vi "Before Run TS.vi"(8 "error in":errorcluster, 11 "Heat Flow Test Stand in":refnum<class "Heat Flow Test Stand.lvclass">) -> (0 "error out":errorcluster, 3 "Heat Flow Test Stand out":refnum<class "Heat Flow Test Stand.lvclass">)   [LabVIEW 2019, in "Test Stands.lvlib" / "Heat Flow Test Stand.lvclass"]
uses:
  Heat Flow Test Stand.lvclass
  C:/Users/wg/Documents/LV_Projects/test-stand/App/Generic Test Stand/Generic Test Stand.lvclass
  DAC/Heat Flow/HeatFlow AIV/DAC HeatFlow AIV.lvclass
  C:/Users/wg/Documents/LV_Projects/test-stand/App/DAC/DAC.lvclass
  Results/Heat Flow Results/Heat Flow Results.lvclass
  Results/Results Method.ctl
  Generic Test Stand/Generic Test Stand.lvclass/Generic Test Stand.ctl
  Heat Flow Test Stand.lvclass/Heat Flow Test Stand.ctl
  DAC/DAC.lvclass/DAC.ctl
  Results/Heat Flow Results/Heat Flow Results.lvclass/Heat Flow Results.ctl
  DAC/DAC.lvclass
  Generic Test Stand/Generic Test Stand.lvclass
  Results/Results.lvlib
  DAC/Heat Flow/RTD Temp/DAC RTD Temp.lvclass
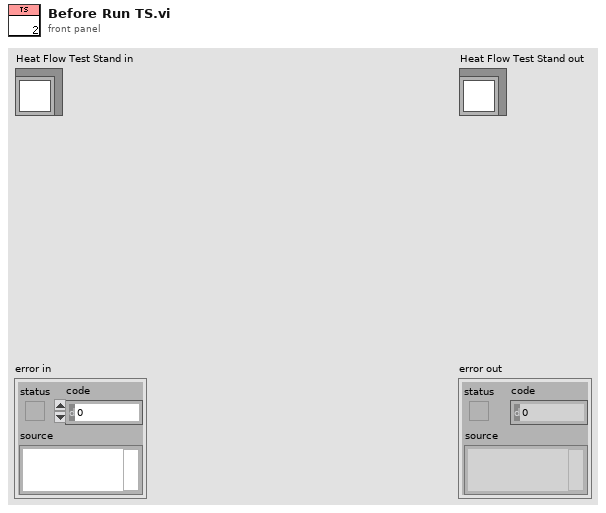
[diagram p1: front panel]
types:
  T1 = typedef "Results.lvlib/Results Method.ctl" = enum16{"Get", "Set"}
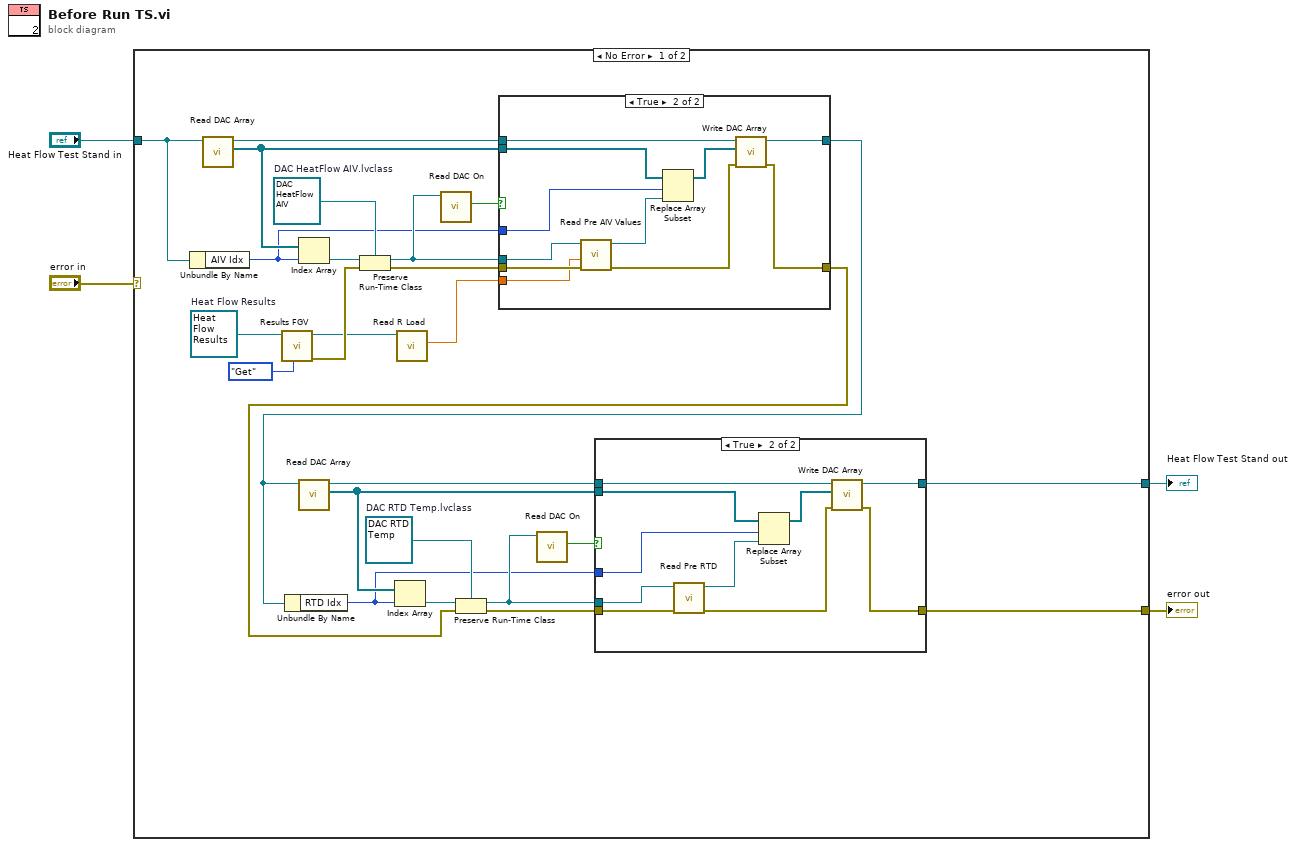
[diagram p0: block diagram]
diagram:
  n1 = case shown="No Error" "error in" {
    selector: "error in" -> [_ w57]
    tunnel: [w7 w57] -> w1
    tunnel: [w8 w56] -> w2
    tunnel: "Heat Flow Test Stand in" -> [w25 w56]
    frame No Error {
      w9 = refnum<class "DAC RTD Temp.lvclass"> refnum  # DAC RTD Temp.lvclass
      w22 = refnum<class "Heat Flow Results.lvclass"> refnum  # Heat Flow Results
      w24 = refnum<class "DAC HeatFlow AIV.lvclass"> refnum  # DAC HeatFlow AIV.lvclass
      n2 = Unbundle By Name(w25) -> ("AIV Idx"=w5:i32)
      n3 = call "Read DAC Array.vi"("Generic Test Stand in"=w25) -> ("DAC Array"=w26:refnum<class "DAC.lvclass">[], "Generic Test Stand out"=w29:refnum<class "Heat Flow Test Stand.lvclass">)  [unwired: 8 in, 1 out]
      n4 = call-dynamic "Results FGV.vi"("Method"=Results_Method."Get", "Results in"=w22) -> ("error out"=w20:errorcluster, "Results out"=w19:refnum<class "Heat Flow Results.lvclass">)  [unwired: 8 in]
      n5 = Index Array(array=w26, index=w5) -> (element=w28:refnum<class "DAC.lvclass">)
      n6 = Preserve Run-Time Class(object in=w28, error in=w20, 2:w24) -> (object out=w23:refnum<class "DAC HeatFlow AIV.lvclass">, error out=w27:errorcluster)
      n7 = call "Read R Load.vi"("Heat Flow Results in"=w19) -> ("R Load"=w18:dbl)  [unwired: 8 in, 2 out]
      n8 = call "Read DAC On.vi"("DAC in"=w23) -> ("DAC On"=w30:bool)  [unwired: 8 in, 2 out]
      n9 = case shown="True" w30 {
        tunnel: w29 -> [w44 w53]
        tunnel: [w44 w55] -> w11
        tunnel: w23 -> [_ w47]
        tunnel: w27 -> [w43 w50]
        tunnel: w26 -> [_ w54]
        tunnel: [w43 w51] -> w10
        tunnel: w18 -> [_ w46]
        tunnel: w5 -> [_ w45]
        frame False {
        }
        frame True {
          n10 = call "Read Pre AIV Values.vi"("error in"=w50, "R Load"=w46, "DAC HeatFlow AIV in"=w47) -> ("error out"=w49:errorcluster, "DAC HeatFlow AIV out"=w48:refnum<class "DAC HeatFlow AIV.lvclass">)  [unwired: 7 in]
          n11 = Replace Array Subset(array=w54, new element=w48, index=w45) -> (w52:refnum<class "DAC.lvclass">[])
          n12 = call "Write DAC Array.vi"("error in (no error)"=w49, "DAC Array"=w52, "Generic Test Stand in"=w53) -> ("error out"=w51:errorcluster, "Generic Test Stand out"=w55:refnum<class "Heat Flow Test Stand.lvclass">)  [unwired: 7 in]
        }
      }
      n13 = Unbundle By Name(w11) -> ("RTD Idx"=w6:i32)
      n14 = call "Read DAC Array.vi"("Generic Test Stand in"=w11) -> ("DAC Array"=w16:refnum<class "DAC.lvclass">[], "Generic Test Stand out"=w13:refnum<class "Heat Flow Test Stand.lvclass">)  [unwired: 8 in, 1 out]
      n15 = Index Array(array=w16, index=w6) -> (element=w14:refnum<class "DAC.lvclass">)
      n16 = Preserve Run-Time Class(object in=w14, error in=w10, 2:w9) -> (object out=w17:refnum<class "DAC RTD Temp.lvclass">, error out=w15:errorcluster)
      n17 = call "Read DAC On.vi"("DAC in"=w17) -> ("DAC On"=w12:bool)  [unwired: 8 in, 2 out]
      n18 = case shown="True" w12 {
        tunnel: w13 -> [w32 w40]
        tunnel: [w32 w42] -> w8
        tunnel: w17 -> [_ w37]
        tunnel: w15 -> [w31 w36]
        tunnel: w16 -> [_ w41]
        tunnel: [w31 w38] -> w7
        tunnel: w6 -> [_ w33]
        frame False {
        }
        frame True {
          n19 = call "Read Pre RTD.vi"("error in"=w36, "DAC RTD Temp in"=w37) -> ("error out"=w34:errorcluster, "DAC RTD Temp out"=w35:refnum<class "DAC RTD Temp.lvclass">)  [unwired: 8 in]
          n20 = Replace Array Subset(array=w41, new element=w35, index=w33) -> (w39:refnum<class "DAC.lvclass">[])
          n21 = call "Write DAC Array.vi"("error in (no error)"=w34, "DAC Array"=w39, "Generic Test Stand in"=w40) -> ("error out"=w38:errorcluster, "Generic Test Stand out"=w42:refnum<class "Heat Flow Test Stand.lvclass">)  [unwired: 7 in]
        }
      }
    }
    frame Error {
    }
  }
  "error out" <- w1
  "Heat Flow Test Stand out" <- w2
